vi "PLL data source -- wrapper.vi"(6 "set-get delay (msec)":i64, 7 "data source action":T2=enum."get", 9 "z  in (V)":cdb, 10 "Freq in (Hz)":dbl=40000.0 format="%#_13g", 11 "PLL data source":T1=enum."SRS865A") -> (1 "z out (V)":cdb=0.00010527635459-2.9308681405e-05i, 2 "Freq out (Hz)":dbl=55115.2, 3 "PLL data source OUT":T1=enum."SRS865A")   [LabVIEW 2018]
uses:
  PLL data source.ctl
  data source action.ctl
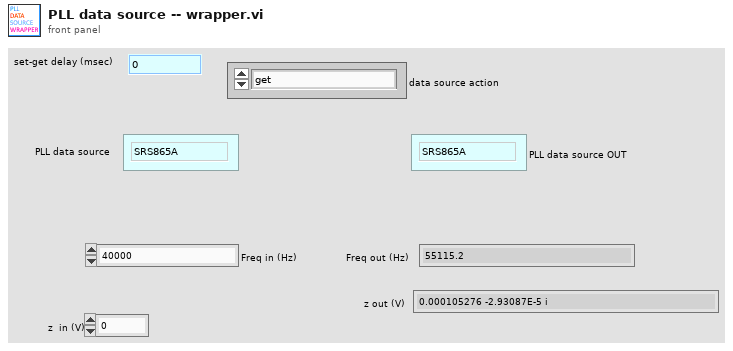
[diagram p1: front panel]
types:
  T1 = typedef "PLL data source.ctl" = enum16{"meta", "MFLI", "SRS865A"}
  T2 = typedef "data source action.ctl" = enum16{"set", "get", "init", "set-and-get"}
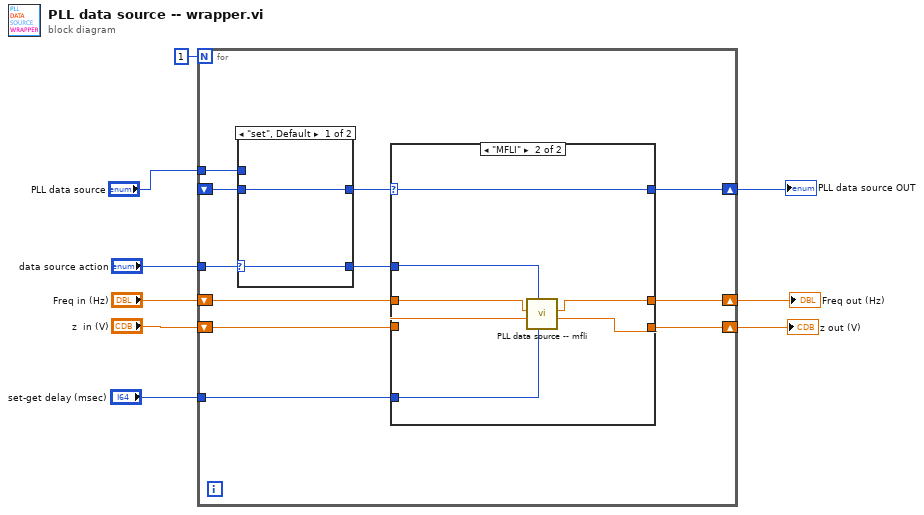
[diagram p0: block diagram]
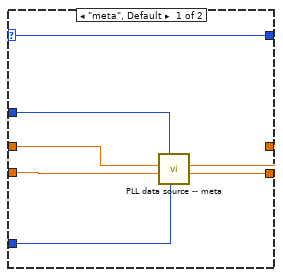
[diagram p3: hidden frame]
diagram:
  n1 = for {
    N: 1 -> [_]
    tunnel: "data source action" -> [w14]
    tunnel: "set-get delay (msec)" -> [w17]
    shift-right: [w18] -> w6
    shift-left: _ -> [w10]
    shift-right: [w20] -> w8
    shift-left: "Freq in (Hz)" -> [w19]
    shift-right: [w15] -> w3
    shift-left: "z  in (V)" -> [w16]
    tunnel: "PLL data source" -> [w12]
    n2 = case shown="\"set\", Default" w14 {
      selector: w14 -> [w21 w24]
      tunnel: [w21 w24] -> w13
      tunnel: w12 -> [_ w23]
      tunnel: [w22 w23] -> w11
      tunnel: w10 -> [w22 _]
      frame "set", Default {
      }
      frame "init" {
      }
    }
    n3 = case shown="\"MFLI\"" w11 {
      selector: w11 -> [w31 w38]
      tunnel: w13 -> [w30 w33]
      tunnel: [w25 w34] -> w20
      tunnel: w19 -> [w28 w37]
      tunnel: [w31 w38] -> w18
      tunnel: w17 -> [w29 w32]
      tunnel: w16 -> [w27 w36]
      tunnel: [w26 w35] -> w15
      frame "meta", Default {
        n4 = call "PLL data source -- meta.vi"("set-get delay (msec)"=w29, "data source action"=w30, "z  in (V)"=w27, "Freq in (Hz)"=w28) -> ("z out (V)"=w26:cdb, "Freq out (Hz)"=w25:dbl)  [unwired: 6 in]
      }
      frame "MFLI" {
        n5 = call "PLL data source -- mfli.vi"("set-get delay (msec)"=w32, "data source action"=w33, "z  in (V)"=w36, "Freq in (Hz)"=w37) -> ("z out (V)"=w35:cdb, "Freq out (Hz)"=w34:dbl)  [unwired: 6 in]
      }
    }
  }
  "Freq out (Hz)" <- w8
  "z out (V)" <- w3
  "PLL data source OUT" <- w6
